vi "Occurrences.vi"() -> ()   [LabVIEW 2022 SP3]
panel:
  out "?":bool
  out "?":bool
  out "?":bool
  out "?":bool
  out "?":bool
  out "?":bool
  out "?":bool
  out "Array 2":string[](array[string])
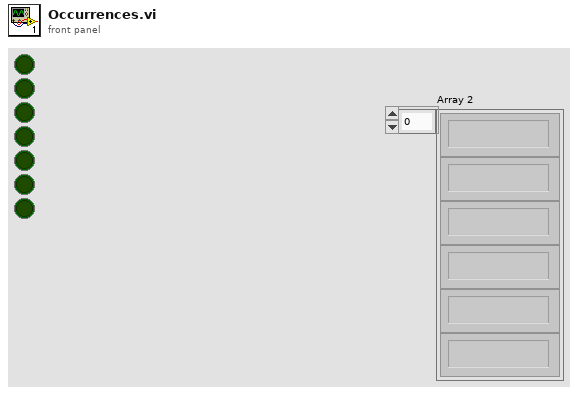
[diagram p1: front panel]
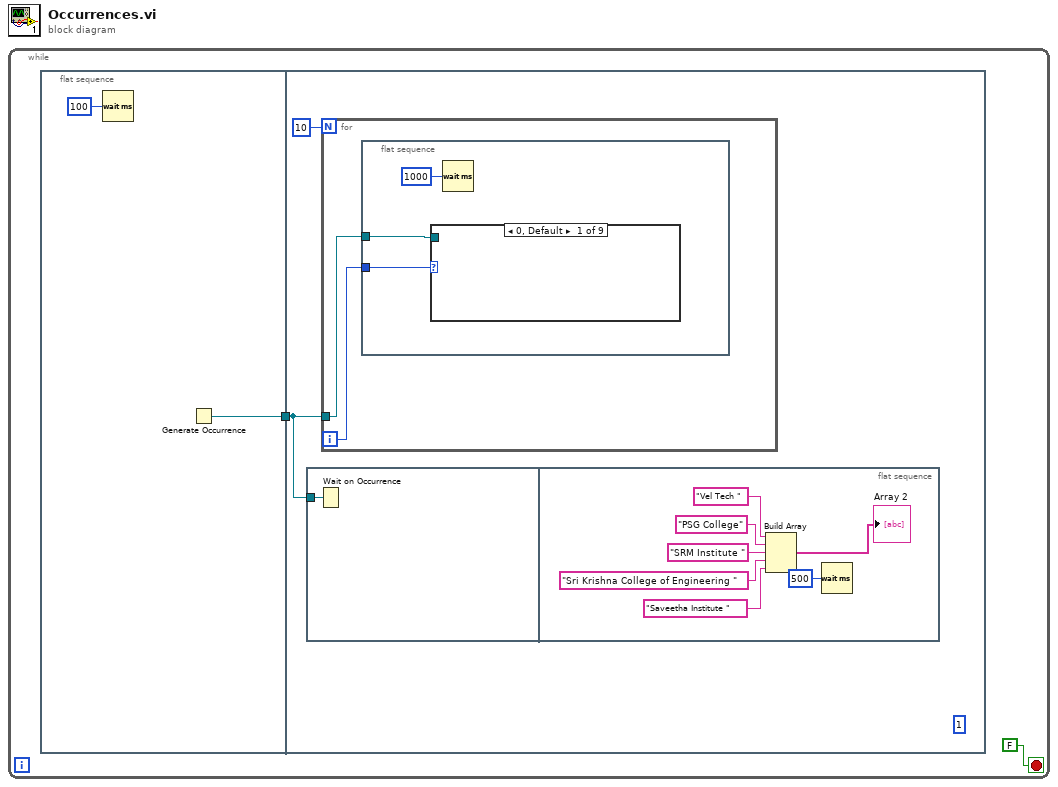
[diagram p0: block diagram]
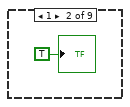
[diagram p2: hidden frame]
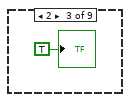
[diagram p3: hidden frame]
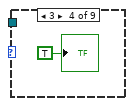
[diagram p4: hidden frame]
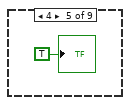
[diagram p5: hidden frame]
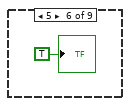
[diagram p6: hidden frame]
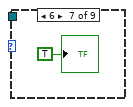
[diagram p7: hidden frame]
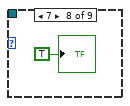
[diagram p8: hidden frame]
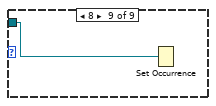
[diagram p9: hidden frame]
diagram:
  n1 = while {
    stop <- FALSE stop-if-true
    n2 = flat-sequence {
      tunnel: [w4] -> w1
      tunnel: w1 -> [w5]
      frame #0 {
        n3 = Wait (ms)(milliseconds to wait=u32 100) -> ()  [unwired: 1 out]
        n4 = Generate Occurrence() -> (w4:refnum<k4>)
      }
      frame #1 {
        (unwired) 1
        n5 = flat-sequence {
          tunnel: w5 -> [w7]
          frame #0 {
            n6 = Wait on Occurrence(2:w7) -> ()  [unwired: 2 in, 1 out]
          }
          frame #1 {
            n7 = Build Array("Vel Tech ", "PSG College", "SRM Institute ", "Sri Krishna College of Engineering ", "Saveetha Institute ") -> (→"Array 2":string[])
            n8 = Wait (ms)(milliseconds to wait=u32 500) -> ()  [unwired: 1 out]
          }
        }
        n9 = for {
          N: 10 -> [_]
          tunnel: w5 -> [w16]
          i -> [w15]
          n10 = flat-sequence {
            tunnel: w16 -> [w17]
            tunnel: w15 -> [w18]
            frame #0 {
              n11 = case shown="0, Default" w18 {
                tunnel: w17 -> [_ _ _ _ _ _ _ _ w27]
                frame 0, Default {
                }
                frame 1 {
                  "?" <- TRUE
                }
                frame 2 {
                  "?" <- TRUE
                }
                frame 3 {
                  "?" <- TRUE
                }
                frame 4 {
                  "?" <- TRUE
                }
                frame 5 {
                  "?" <- TRUE
                }
                frame 6 {
                  "?" <- TRUE
                }
                frame 7 {
                  "?" <- TRUE
                }
                frame 8 {
                  n12 = Set Occurrence(w27) -> ()
                }
              }
              n13 = Wait (ms)(milliseconds to wait=u32 1000) -> ()  [unwired: 1 out]
            }
          }
        }
      }
    }
  }
